vi "projekt 1 (SubVI).vi"(0 "Temp F":dbl, 9 "Boolean":bool) -> (14 "Numeric Control":dbl)   [LabVIEW 2017]
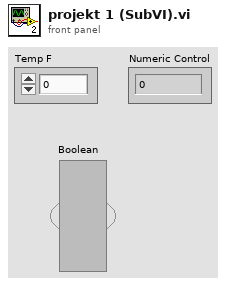
[diagram p1: front panel]
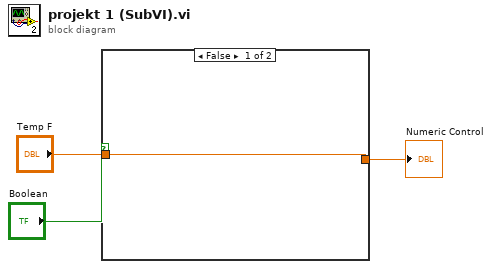
[diagram p0: block diagram]
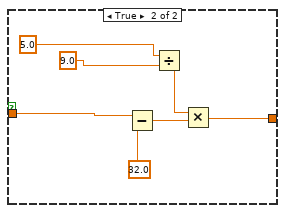
[diagram p2: hidden frame]
diagram:
  n1 = case shown="False" "Boolean" {
    tunnel: [w4 w7] -> w3
    tunnel: "Temp F" -> [w4 w5]
    frame False {
    }
    frame True {
      n2 = Subtract(x=w5, y=32.0 ("x-y")) -> (x-y=w6:dbl)
      n3 = Divide(x=5.0 ("y"), y=9.0 ("x/y")) -> (x/y=w8:dbl)
      n4 = Multiply(x=w8, y=w6) -> (x*y=w7:dbl)
    }
  }
  "Numeric Control" <- w3
